vi "KtFilterHPF (SubVI).vi"(9 "frq":dbl, 10 "HPFFilterNum":T1(ring), 11 "Array":cluster{"Frq":dbl[], "Kt":dbl[]}[](array[cluster])) -> (3 "Numeric":dbl)   [LabVIEW 2017]
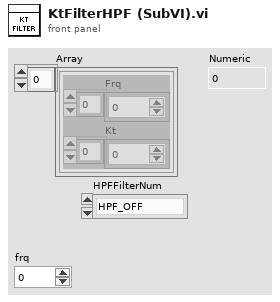
[diagram p1: front panel]
types:
  T1 = enum16{"HPF_OFF", "1", "2", "3", "4", "5", "6", "7", "8", "9", "10"}
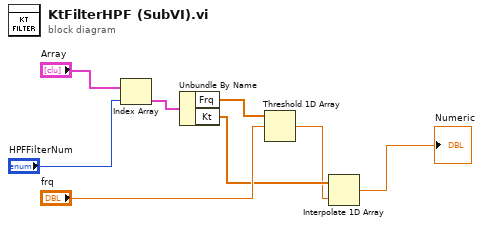
[diagram p0: block diagram]
diagram:
  n1 = Index Array(array="Array", index="HPFFilterNum") -> (element=w5:cluster{"Frq":dbl[], "Kt":dbl[]})
  n2 = Unbundle By Name(w5) -> ("Frq"=w6:dbl[], "Kt"=w7:dbl[])
  n3 = Threshold 1D Array(2:"frq", 3:w6) -> (0:w2:dbl)  [unwired: 1 in]
  n4 = Interpolate 1D Array(1:w2, 2:w7) -> (0:→"Numeric":dbl)
